vi "ClearBD.vi"(8 "error in":errorcluster, 11 "reference":refnum<vi>) -> (0 "error out":errorcluster, 3 "reference out":refnum<vi>)   [LabVIEW 2013, in "data interface script.lvlib"]
uses:
  data interface script.lvlib
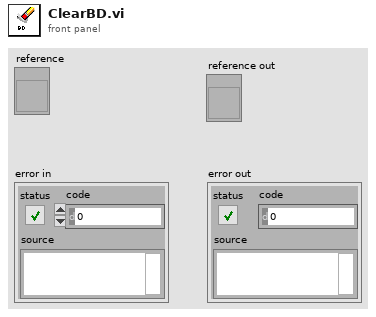
[diagram p1: front panel]
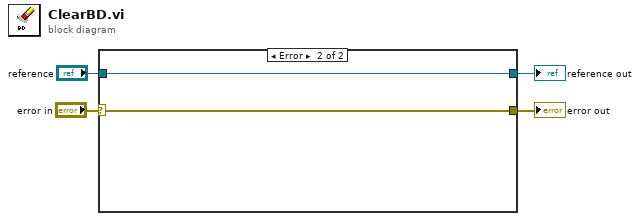
[diagram p0: block diagram]
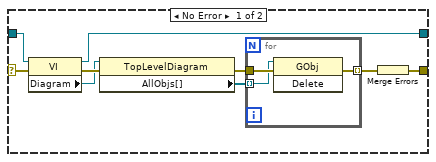
[diagram p2: hidden frame]
diagram:
  n1 = case shown="Error" "error in" {
    selector: "error in" -> [w5 w17]
    tunnel: "reference" -> [w8 w18]
    tunnel: [w7 w18] -> w3
    tunnel: [w6 w17] -> w2
    frame No Error {
      n2 = property class="VI"(reference=w8, error in=w5) -> (reference out=w7:refnum<vi>, error out=w13:errorcluster, "Diagram"=w12:refnum<vi>)
      n3 = property class="TopLevelDiagram"(reference=w12, error in=w13) -> (error out=w11:errorcluster, "AllObjs[]"=w10:refnum<vi>[])  [unwired: 1 out]
      n4 = for {
        tunnel: w11 -> [w16]
        tunnel: w10 -> [w15] mode=indexing
        tunnel: [w14] -> w9 mode=indexing
        n5 = invoke class="GObj" method="Delete"(reference=w15, error in=w16) -> (error out=w14:errorcluster)  [unwired: 1 in, 2 out]
      }
      n6 = Merge Errors(w9) -> (w6:errorcluster)
    }
    frame Error {
    }
  }
  "reference out" <- w3
  "error out" <- w2
